vi "omni drive gyro.vi"(0 "Drive RefNum":T3={"DevStatus"={"status"=FALSE, "code"=0, "source"=""}, "Motors[]"=[], "Square Inputs"=FALSE, "Max Output"=1.0}, 1 "X Axis":dbl, 2 "Y Axis":dbl, 3 "Z Axis":dbl, 4 "Drive Mode":T1=enum."Arcade Drive", 5 "Center Motor":T4={"DeviceStatus"={"status"=FALSE, "code"=0, "source"=""}, "Type"=enum."PWM", "PWM"={"Controller"=enum."Controller 1", "PWM Channel"=enum."Invalid", "DeadBand"={"Name"="", "maxPositivePwm"=0, "minPositivePwm"=0, "centerPwm"=0, "maxNegativePwm"=0, "minNegativePwm"=0, "angularRange"=0}}, "CAN"={"Device Number"=0, "Control Mode"=enum."Percent VBus", "Semaphore"=refnum, "Max Vout"=12.0, "TalonSRX Control Mode"=enum."Percent VBus"}, "Invert"=FALSE, "TransformRef"=refnum, "InvTransformRef"=refnum}, 9 "Desired Angle":dbl) -> ()   [LabVIEW 2014]
uses:
  typedefs/drive mode.ctl
  <vilib>/Rock Robotics/WPI/RobotDrive/WPI_RobotDriveDevRef.ctl
  <vilib>/Rock Robotics/WPI/MotorControl/WPI_MotorControlDeviceRef.ctl
  <vilib>/Rock Robotics/WPI/MotorControl/WPI_MotorControlType.ctl
  <vilib>/Rock Robotics/SystemInterfaces/Typedef/FPGA_TypedefDigitalModule.ctl
  <vilib>/Rock Robotics/SystemInterfaces/DIO/FPGA_DIOPWMChannel.ctl
  <vilib>/Rock Robotics/WPI/PWM/WPI_PWMDeadband.ctl
  <vilib>/Rock Robotics/WPI/CAN/Jaguar/SubVIs/WPI_CANJaguar_ControlMode.ctl
  <vilib>/Rock Robotics/WPI/CAN/TalonSRX/WPI_CANTalonSRX_APIControlMode.ctl
  <vilib>/Rock Robotics/WPI/PWM/WPI_PWMTransform_ConPane.ctl
  typedefs/state machine/subStates.ctl
  global variables/devrefs.vi
  <vilib>/addons/control/pid/pid.llb/PID (DBL).vi
  <vilib>/Rock Robotics/WPI/RobotDrive/WPI_RobotDriveArcadeDrive_Standard(NoSaturation).vi
  global variables/dashboard data.vi
  <vilib>/addons/control/pid/NI_PID_pid.lvlib
panel:
  in  "Omni-Drive Tab Control":enum32{"Drive I/O", "PID", "Motor Controls"}(tab)
  in  "Spin Factor":dbl(slide) min=0.0 max=2.0 step=0.1 scale=0.0..2.0
  in  "PID Gains":T2={"proportional gain (Kc)"=0.0592, "integral time (Ti, min)"=0.0015, "derivative time (Td, min)"=0.0025} {"derivative time (Td, min)" step=0.0001 format="%.5f"; "integral time (Ti, min)" step=0.0001 format="%.5f"; "proportional gain (Kc)" step=0.0001 format="%.5f"}
  out "Gyro Temp °C":dbl
  out "Gyro Temp °F":dbl
  out "Setpoint Angle":dbl format="%#_6g°"
  out "Current Angle":dbl format="%#_g°"
  out "PID & Gyro Waveform Chart":cluster{"Angle":dbl, "output":dbl}(graph)
  out "Angular Rate":dbl
  # "Drive the Robot in Either Arcade Style or H-Drive Style"
  # "VI Inputs"
  # "OKish values rev1\nP: 0.00040\nI: 0.00100\nD: 0.00000\n\nPretty Good values\nP: 0.02\nI: 0.005\nD: 0.001\n\nBetter values?\nP: 0.0025\nI: 0.002\nD: 0.001\n\n0.009\n0.006"
  # "Thats a type def so you can't change it to the system\ncontrol otherwise it will no longer by linked to the typedef,\nand you can't re-link it"
  # "Temporary"
  # "Does this empty space make you feel uncomfortable?"
  # "Yes."
  # "I'm glad you feel that way."
  # "Note: Current Angle only updated in H-Drive, \nSetpoint updated in Arcade"
  # "°/sec"
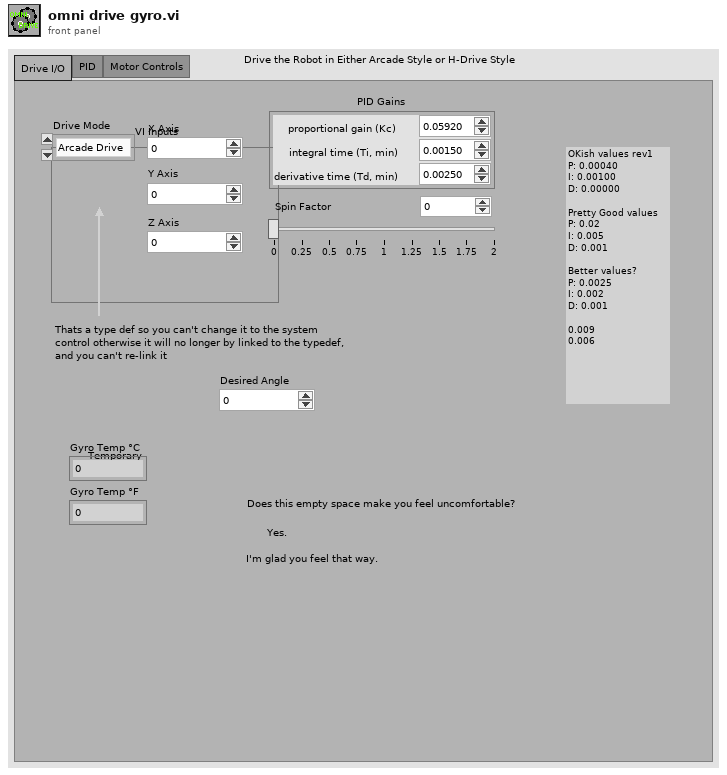
[diagram p1: front panel]
types:
  T1 = typedef "drive mode.ctl" = enum16{"Left/Right X/Y Control", "Arcade Drive", "H-Drive", "H-Drive Spin", "H-Drive PID", "Autonomous"}
  T2 = cluster{"proportional gain (Kc)":dbl, "integral time (Ti, min)":dbl, "derivative time (Td, min)":dbl}
  T3 = typedef "WPI_RobotDriveDevRef.ctl" = cluster{"DevStatus":errorcluster, "Motors[]":T4[], "Square Inputs":bool, "Max Output":dbl}
  T4 = typedef "WPI_MotorControlDeviceRef.ctl" = cluster{"DeviceStatus":errorcluster, "Type":T5, "PWM":cluster{"Controller":T6, "PWM Channel":T7, "DeadBand":T8}, "CAN":cluster{"Device Number":u8, "Control Mode":T9, "Semaphore":T10, "Max Vout":dbl, "TalonSRX Control Mode":T11}, "Invert":bool, "TransformRef":T12, "InvTransformRef":T12}
  T5 = typedef "WPI_MotorControlType.ctl" = enum16{"PWM", "CAN", "CANTalonSRX"}
  T6 = typedef "FPGA_TypedefDigitalModule.ctl" = enum16{"Controller 1"}
  T7 = typedef "FPGA_DIOPWMChannel.ctl" = enum8{"PWM 0", "PWM 1", "PWM 2", "PWM 3", "PWM 4", "PWM 5", "PWM 6", "PWM 7", "PWM 8", "PWM 9", "PWM MXP 0", "PWM MXP 1", "PWM MXP 2", "PWM MXP 3", "PWM MXP 4", "PWM MXP 5", "PWM MXP 6", "PWM MXP 7", "PWM MXP 8", "PWM MXP 9", "Invalid"}
  T8 = typedef "WPI_PWMDeadband.ctl" = cluster{"Name":string, "maxPositivePwm":i32, "minPositivePwm":i32, "centerPwm":i32, "maxNegativePwm":i32, "minNegativePwm":i32, "angularRange":u16}
  T9 = typedef "WPI_CANJaguar_ControlMode.ctl" = enum8{"Percent VBus", "Current", "Speed", "Position", "Voltage"}
  T10 = typedef "Semaphore RefNum" = refnum<k1>
  T11 = typedef "WPI_CANTalonSRX_APIControlMode.ctl" = enum8{"Percent VBus", "Speed", "Position", "Slave", "Unchanged / Invalid"}
  T12 = typedef "WPI_PWMTransform_ConPane.ctl" = refnum<vi>
  T13 = typedef "subStates.ctl" = enum16{"null", "wait", "driver control", "auto", "manual override", "hold position", "rotate", "test", "end"}
  T14 = typedef "WPI_GyroDevRef.ctl" = cluster{"DevStatus":errorcluster, "Analog Module":T15, "Analog Channel":T16, "Offset":dbl, "Gain (VoltsPerDegree/Second)":dbl}
  T15 = typedef "FPGA_TypedefAnalogModule.ctl" = enum16{"Controller 1"}
  T16 = typedef "FPGA_AIChannel.ctl" = enum8{"AI 0", "AI 1", "AI 2", "AI 3", "AI MXP 0", "AI MXP 1", "AI MXP 2", "AI MXP 3", "Invalid"}
  T17 = typedef "WPI_AnalogChannelDevRef.ctl" = cluster{"DevStatus":errorcluster, "Controller":T15, "Analog Channel":T16}
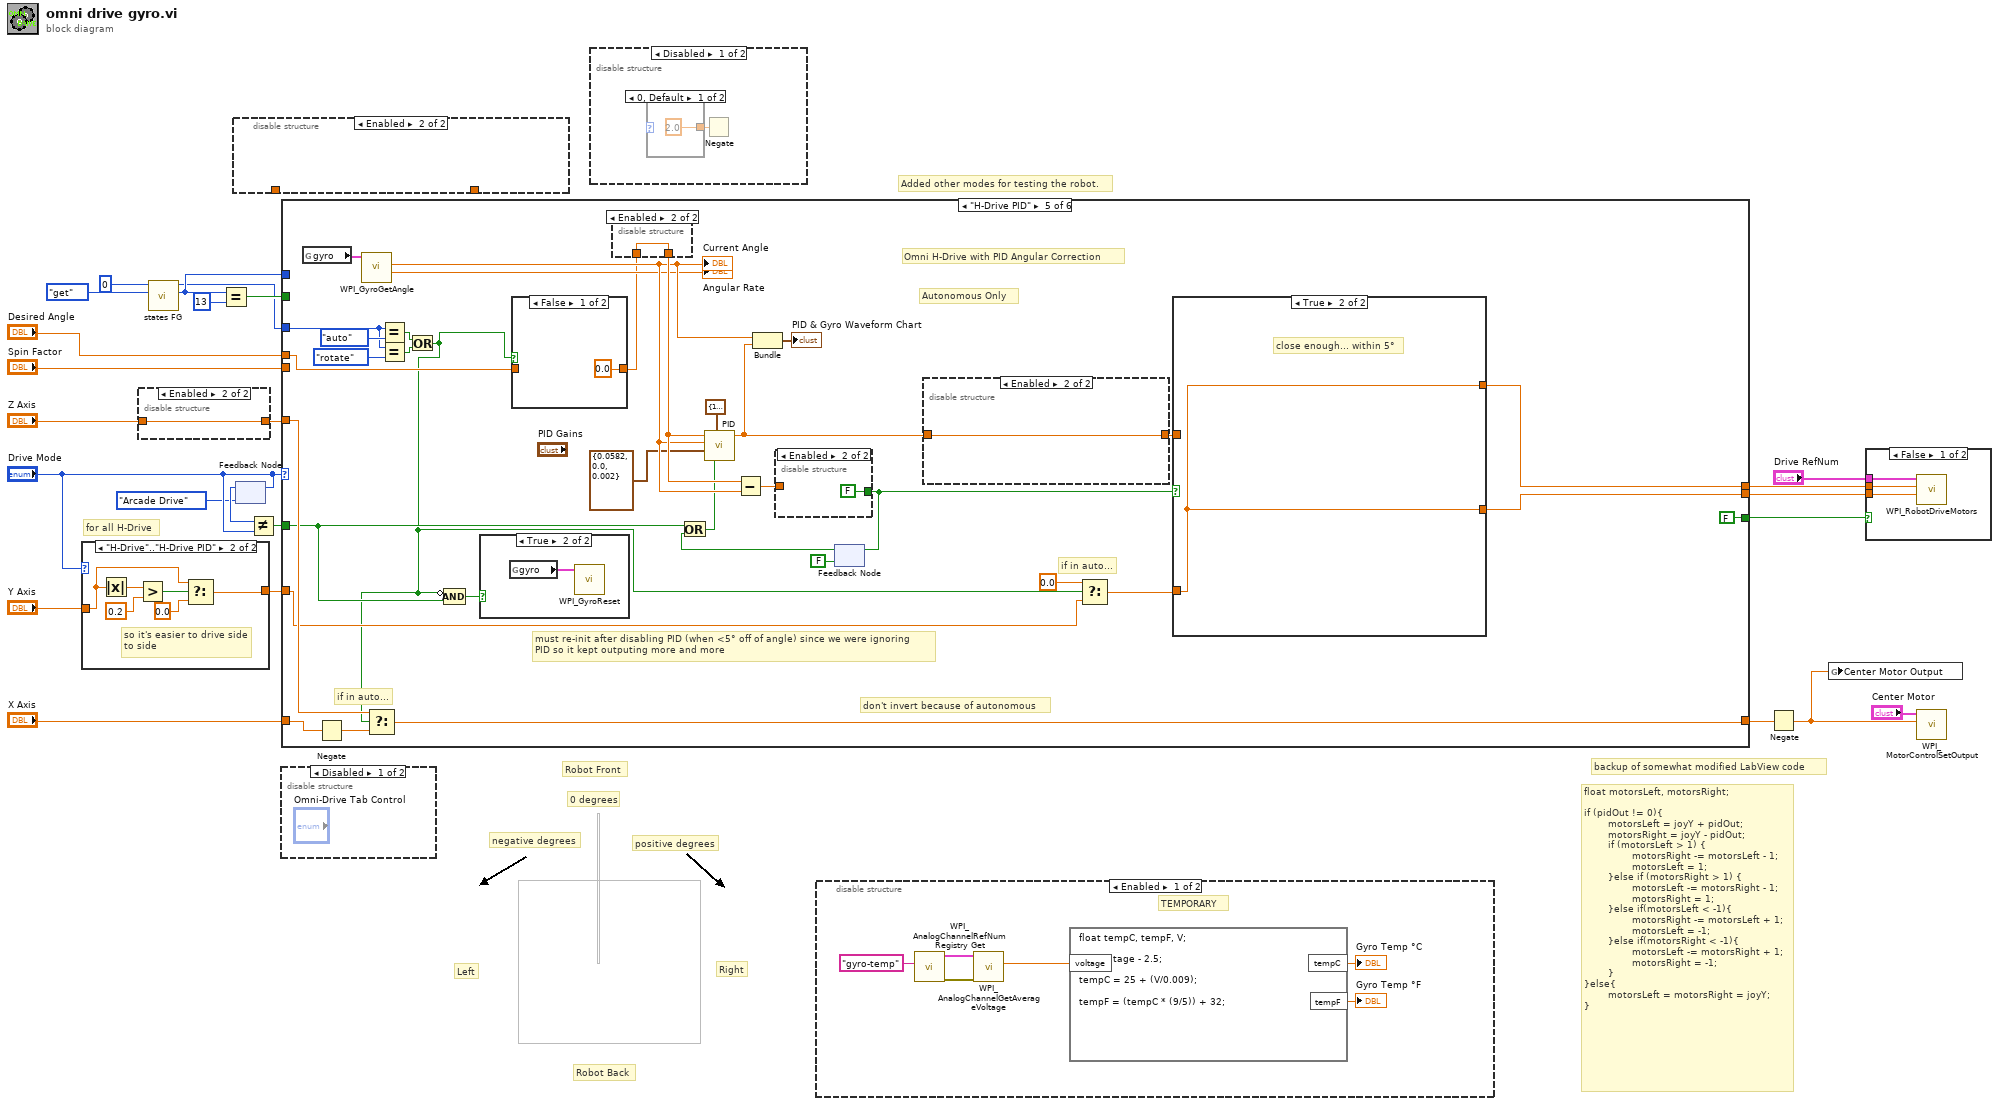
[diagram p0: block diagram]
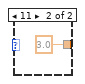
[diagram p2: hidden frame]
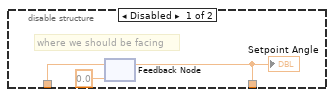
[diagram p4: hidden frame]
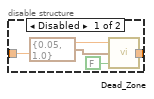
[diagram p7: hidden frame]
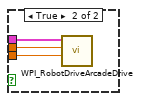
[diagram p9: hidden frame]
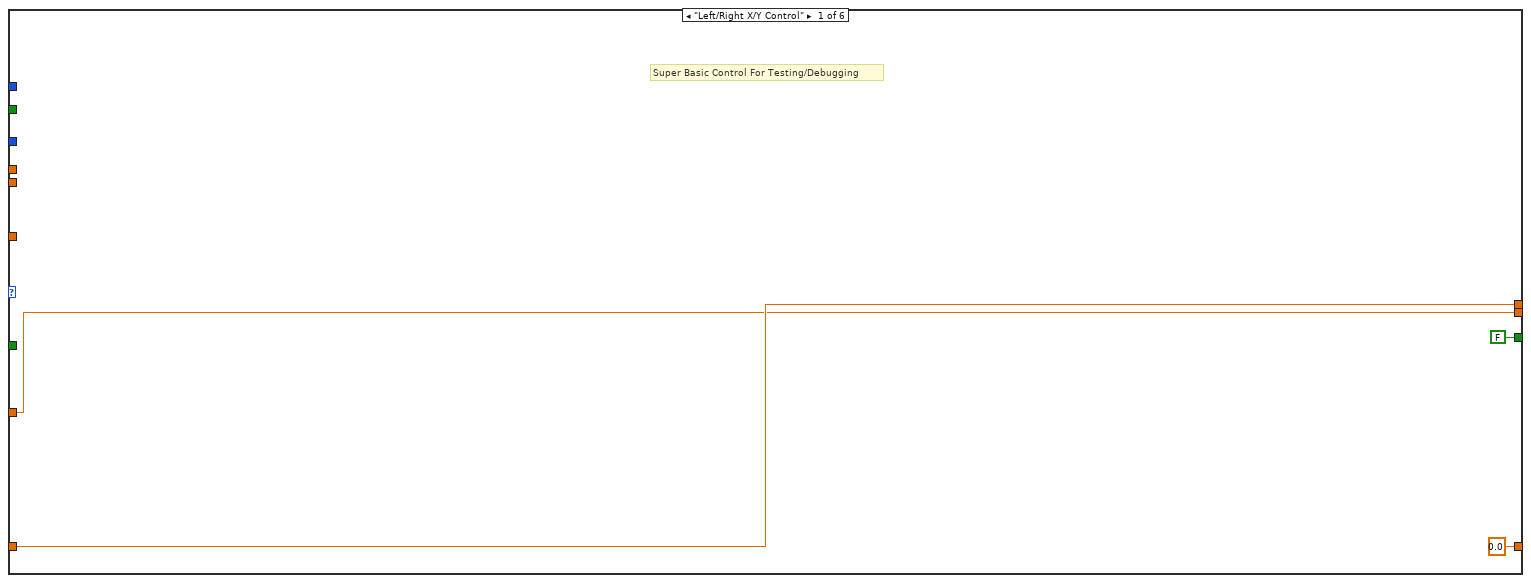
[diagram p10: hidden frame]
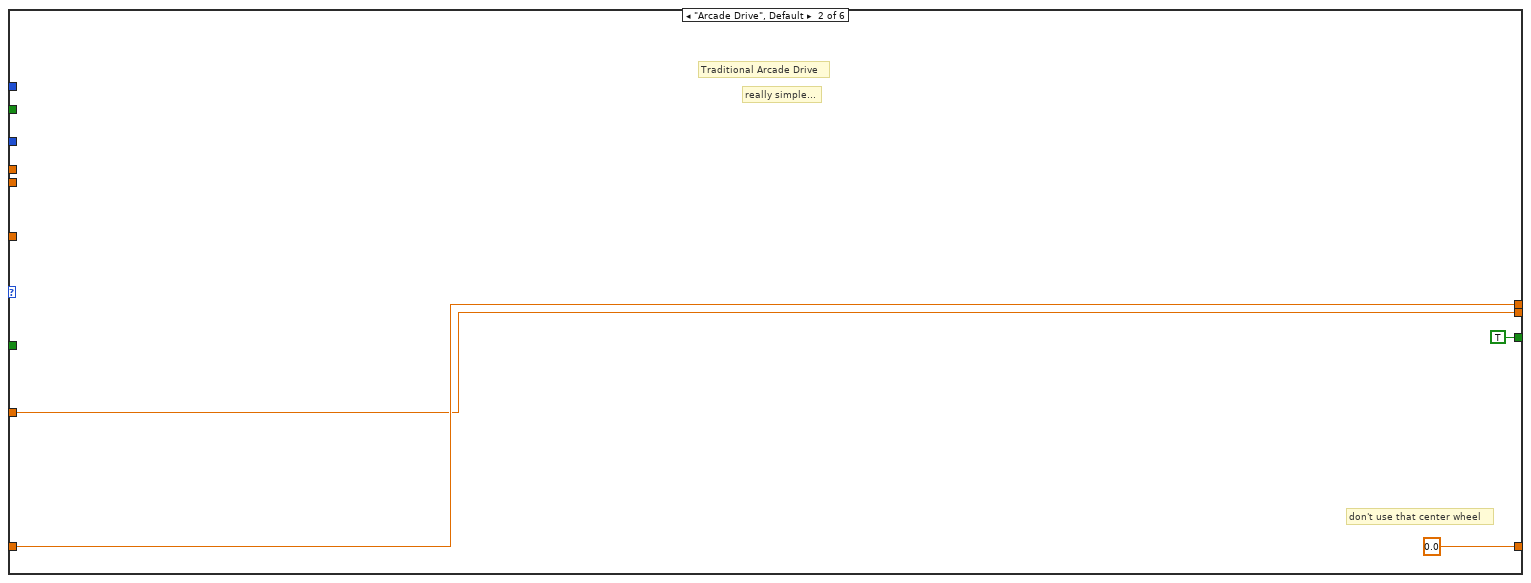
[diagram p11: hidden frame]
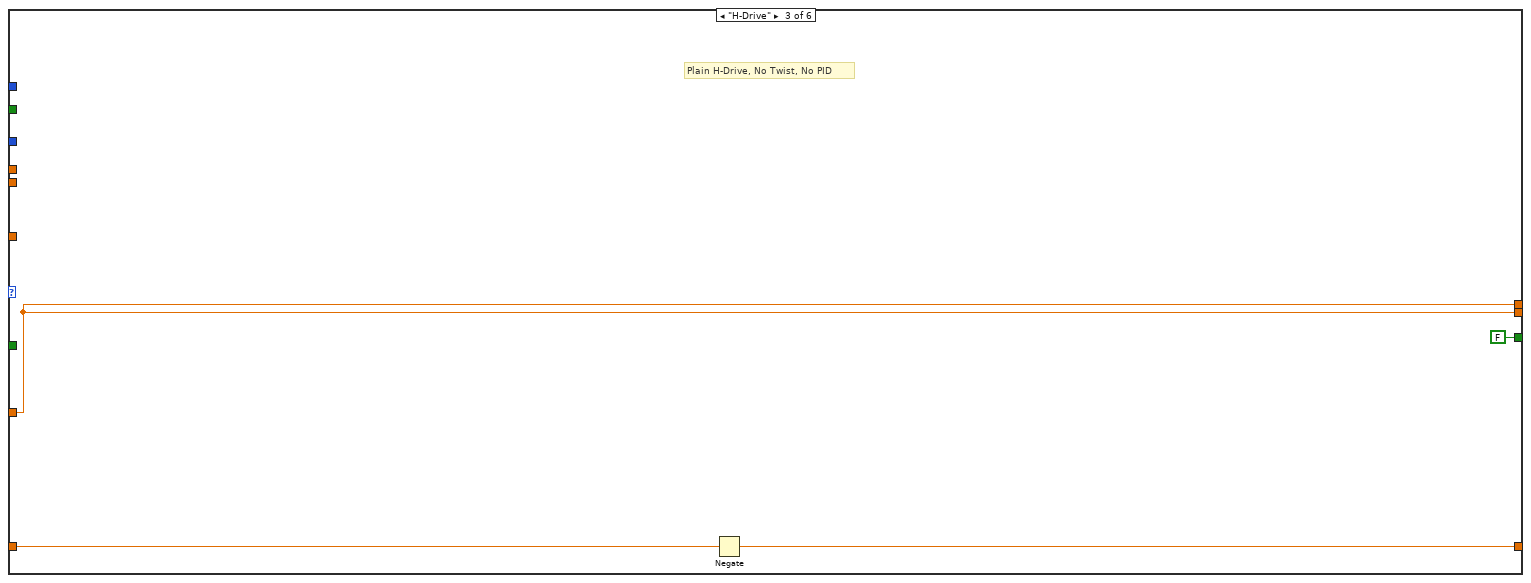
[diagram p12: hidden frame]
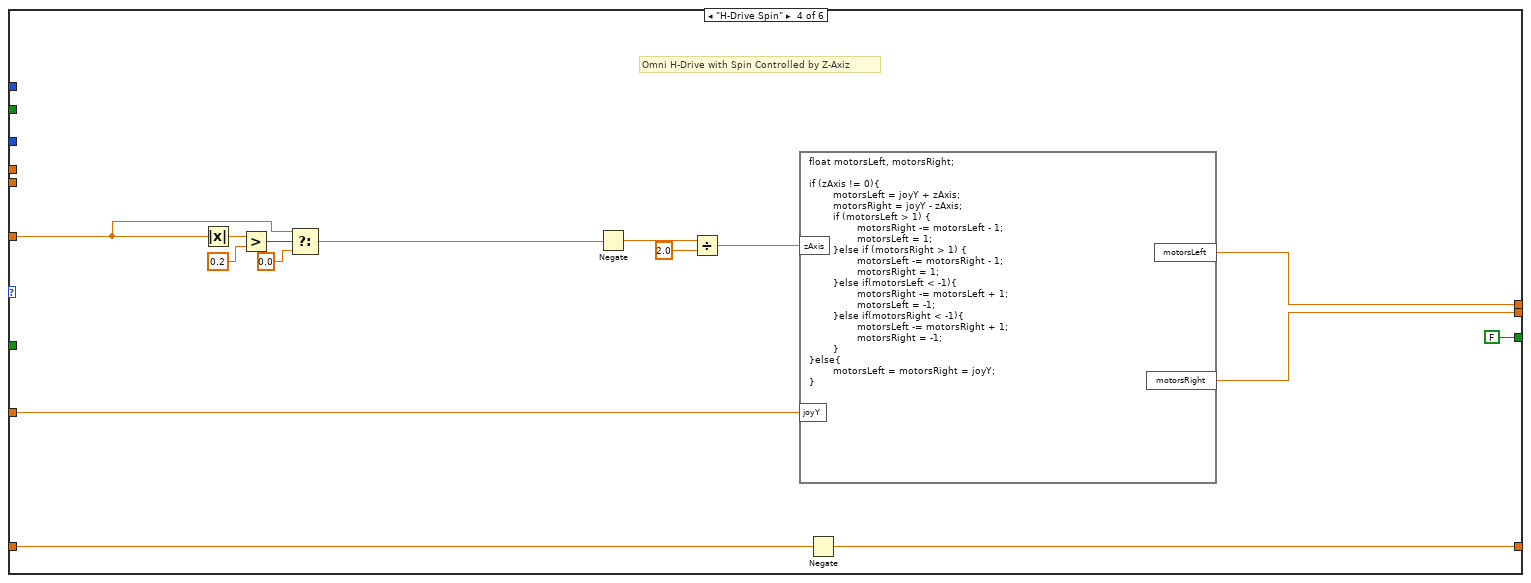
[diagram p13: hidden frame]
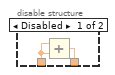
[diagram p14: hidden frame]
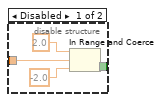
[diagram p17: hidden frame]
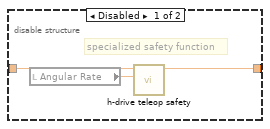
[diagram p18: hidden frame]
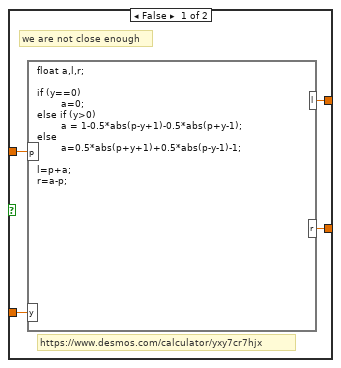
[diagram p19: hidden frame]
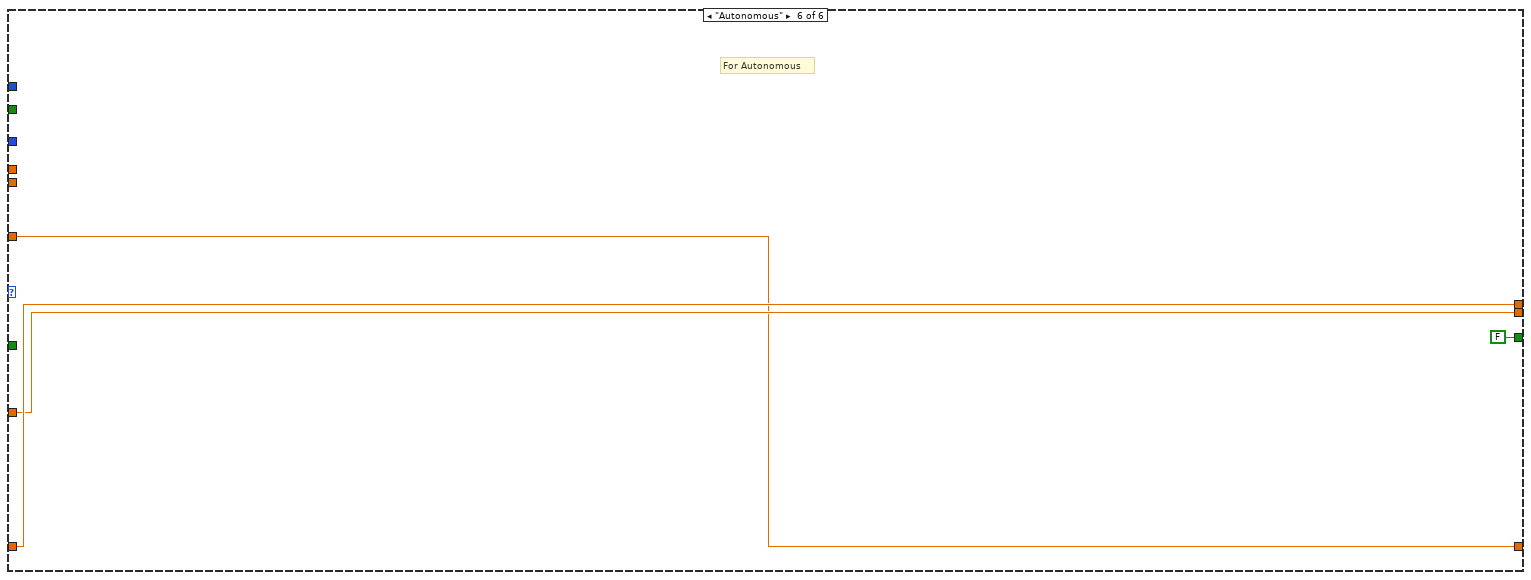
[diagram p20: hidden frame]
diagram:
  # "for all H-Drive"
  # "Added other modes for testing the robot."
  # "backup of somewhat modified LabView code"
  # "float motorsLeft, motorsRight;\n\nif (pidOut != 0){\n        motorsLeft = joyY + pidOut;\n        motorsRight = joyY - pidOut;\n        if (motorsLeft > 1) {\n                motorsRight -= motorsLeft - 1;\n                motorsLeft = 1;\n        }else if (motorsRight > 1) {\n                motorsLeft -= motorsRight - 1;\n                motorsRight = 1;\n        }else if(motorsLeft < -1){\n                motorsRight -= motorsLeft + 1;\n                motorsLeft = -1;\n        }else if(motorsRight < -1){\n                motorsLeft -= motorsRight + 1;\n                motorsRight = -1;\n        }\n}else{\n        motorsLeft = motorsRight = joyY;\n}"
  # "Robot Back"
  # "Right"
  # "Left"
  # "negative degrees"
  # "positive degrees"
  # "0 degrees"
  # "Robot Front"
  n1 = case shown="\"H-Drive\"..\"H-Drive PID\"" "Drive Mode" {
    tunnel: [w25 w26] -> w11
    tunnel: "Y Axis" -> [w25 w28]
    frame Default {
    }
    frame "H-Drive".."H-Drive PID" {
      # "so it's easier to drive side\nto side"
      n2 = Absolute Value(x=w28) -> (abs(x)=w31:dbl)
      n3 = Greater?(x=w31, y=0.2) -> (0:w29:bool)
      n4 = Select(t=w28, s=w29, f=0.0) -> (s? t:f=w26:dbl)
    }
  }
  n5 = disable-structure shown="Enabled" {
    disable-tunnel: [w35 w36] -> w13
    disable-tunnel: "Z Axis" -> [w34 w36]
    frame Disabled {
      n6 = call "Dead_Zone.vi"("Slope of 1"=FALSE, "Dead Zone and Limits"=cluster{dbl, dbl} {0.05, 1.0}, "Input"=w34) -> ("Output"=w35:dbl)  [unwired: 1 in]
    }
    frame Enabled {
    }
  }
  n7 = call "states FG.vi"("menu (get)"=enum16{"set", "get"}."get", "Loop ID"=0) -> ("state # out"=w3:i32, "subState out"=w2:T13)  [unwired: 6 in, 2 out]
  n8 = Equal?(x=w3, y=13) -> (x = y?=w5:bool)
  n9 = disable-structure shown="Enabled" {
    disable-tunnel: _ -> [w39 _]
    disable-tunnel: [w37 _] -> _
    frame Disabled {
      # "where we should be facing"
      n10 = feedback #1(0.0) -> (w37:dbl)
      n11 = feedback-in #1(w39) -> ()
      "Setpoint Angle" <- w39
    }
    frame Enabled {
    }
  }
  n12 = feedback-in #2("Drive Mode") -> ()
  n13 = feedback #2(drive_mode."Arcade Drive" ("Drive Mode")) -> (w17:T1)
  n14 = Not Equal?(x=w17, y="Drive Mode") -> (x != y?=w16:bool)
  n15 = case shown="\"H-Drive PID\"" "Drive Mode" {
    tunnel: [0.0 ("X Axis") 0.0 w48 w58 w79 w121] -> w14
    tunnel: [w42 w46 w50 w62 w85 w122] -> w23
    tunnel: [w43 w47 w50 w63 w86 w123] -> w22
    tunnel: "X Axis" -> [w43 w47 w49 w64 w78 w123]
    tunnel: w11 -> [w42 w46 w50 w65 w75 w122]
    tunnel: [FALSE TRUE FALSE FALSE FALSE FALSE] -> w20
    tunnel: w16 -> [_ _ _ _ w81 _]
    tunnel: w13 -> [_ _ _ w52 w82 w121]
    tunnel: "Spin Factor" -> [_ _ _ _ _ _]
    tunnel: w5 -> [_ _ _ _ _ _]
    tunnel: w3 -> [_ _ _ _ _ _]
    tunnel: w2 -> [_ _ _ _ w71 _]
    tunnel: "Desired Angle" -> [_ _ _ _ w74 _]
    frame "Left/Right X/Y Control" {
      # "Super Basic Control For Testing/Debugging"
    }
    frame "Arcade Drive", Default {
      # "really simple..."
      # "don't use that center wheel"
      # "Traditional Arcade Drive"
    }
    frame "H-Drive" {
      # "Plain H-Drive, No Twist, No PID"
      n16 = Negate(x=w49) -> (-x=w48:dbl)
    }
    frame "H-Drive Spin" {
      # "Omni H-Drive with Spin Controlled by Z-Axiz"
      n17 = Absolute Value(x=w52) -> (abs(x)=w54:dbl)
      n18 = Greater?(x=w54, y=0.2) -> (0:w56:bool)
      n19 = Select(t=w52, s=w56, f=0.0) -> (s? t:f=w53:dbl)
      n20 = Negate(x=w53) -> (-x=w59:dbl)
      n21 = Divide(x=w59, y=2.0 ("x")) -> (x/y=w61:dbl)
      n22 = formula code="float motorsLeft, motorsRight;\n\nif (zAxis != 0){\n        motorsLeft = joyY + zAxis;\n        motorsRight = joyY - zAxis;\n        if (motorsLeft > 1) {\n                motorsRight -= motorsLeft - 1;\n                motorsLeft = 1;\n        }else if (motorsRight > 1) {\n                motorsLeft -= motorsRight - 1;\n                motorsRight = 1;\n        }else if(motorsLeft < -1){\n                motorsRight -= motorsLeft + 1;\n                motorsLeft = -1;\n        }else if(motorsRight < -1){\n                motorsLeft -= motorsRight + 1;\n                motorsRight = -1;\n        }\n}else{\n        motorsLeft = motorsRight = joyY;\n}"("zAxis"=w61, "joyY"=w65) -> ("motorsLeft"=w63:dbl, "motorsRight"=w62:dbl)
      n23 = Negate(x=w64) -> (-x=w58:dbl)
    }
    frame "H-Drive PID" {
      # "if in auto..."
      # "if in auto..."
      # "don't invert because of autonomous"
      # "Autonomous Only"
      # "must re-init after disabling PID (when <5° off of angle) since we were ignoring\nPID so it kept outputing more and more"
      # "Omni H-Drive with PID Angular Correction"
      n24 = global read "devrefs.vi" "gyro"() -> (w96:T14)
      n25 = Negate(x=w78) -> (-x=w67:dbl)
      n26 = call <vilib>:"WPI_GyroGetAngle.vi"("GyroDevRef"=w96) -> ("Angular Rate"=→"Angular Rate":dbl, "Angle"=w99:dbl)  [unwired: 7 in, 2 out]
      "Current Angle" <- w99
      n27 = Equal?(x=w71, y=subStates."auto") -> (x = y?=w69:bool)
      n28 = Equal?(x=w71, y=subStates."rotate") -> (x = y?=w70:bool)
      n29 = Or(x=w69, y=w70) -> (x .or. y?=w68:bool)
      n30 = Select(t=w82, s=w68, f=w67) -> (s? t:f=w79:dbl)
      n31 = Compound Arithmetic op=AND(invert w68, w81) -> (w80:bool)
      n32 = case shown="True" w80 {
        frame False {
        }
        frame True {
          n33 = global read "devrefs.vi" "gyro"() -> (w104:T14)
          n34 = call <vilib>:"WPI_GyroReset.vi"("GyroDevRef"=w104) -> ()  [unwired: 9 in, 2 out]
        }
      }
      n35 = case shown="False" w68 {
        tunnel: [0.0 w106] -> w84
        tunnel: w74 -> [_ w106]
        frame False {
        }
        frame True {
        }
      }
      n36 = disable-structure shown="Enabled" {
        disable-tunnel: [w102 w103] -> w100
        disable-tunnel: w84 -> [w101 w103]
        frame Disabled {
          n37 = Add(x=w101, y=w101) -> (x+y=w102:dbl)
        }
        frame Enabled {
        }
      }
      n38 = Subtract(x=w100, y=w99) -> (x-y=w91:dbl)
      n39 = disable-structure shown="Enabled" {
        disable-tunnel: [w110 FALSE] -> w94
        disable-tunnel: w91 -> [w109 _]
        frame Disabled {
          n40 = In Range and Coerce(upper limit=2.0, x=w109, lower limit=-2.0 ("upper limit")) -> (In Range?=w110:bool)  [unwired: 1 out]
        }
        frame Enabled {
        }
      }
      n41 = feedback #3(FALSE) -> (w90:bool)
      n42 = Or(x=w81, y=w90) -> (x .or. y?=w93:bool)
      n43 = call-poly <vilib>:"PID.vi"("reinitialize? (F)"=w93, "output range"=cluster{"output high":dbl, "output low":dbl} {"output high"=1.0, "output low"=-1.0}, "PID gains"=T2 {"proportional gain (Kc)"=0.0582, "integral time (Ti, min)"=0.0, "derivative time (Td, min)"=0.002} ("PID Gains 2"), "process variable"=w99, "setpoint"=w100) -> ("output"=w88:dbl)  [unwired: 5 in, 1 out]
      n44 = Bundle("Angle"=w99, "output"=w88) -> (→"PID & Gyro Waveform Chart":cluster{"Angle":dbl, "output":dbl})  [unwired: 1 in]
      n45 = feedback-in #3(w94) -> ()
      n46 = disable-structure shown="Enabled" {
        disable-tunnel: w88 -> [w114 w115]
        disable-tunnel: [w113 w115] -> w87
        frame Disabled {
          # "specialized safety function"
          n47 = local read "Angular Rate"() -> (w112:dbl)
          n48 = call "h-drive teleop safety.vi"("Gyro Angular Rate"=w112, "Input"=w114) -> ("Output"=w113:dbl)  [unwired: 9 in]
        }
        frame Enabled {
        }
      }
      n49 = Select(t=0.0, s=w68, f=w75) -> (s? t:f=w77:dbl)
      n50 = case shown="True" w94 {
        tunnel: w87 -> [w117 _]
        tunnel: [w119 w120] -> w85
        tunnel: [w118 w120] -> w86
        tunnel: w77 -> [w116 w120]
        frame False {
          # "https://www.desmos.com/calculator/yxy7cr7hjx"
          # "we are not close enough"
          n51 = formula code="float a,l,r;\n\nif (y==0) \n        a=0;\nelse if (y>0) \n        a = 1-0.5*abs(p-y+1)-0.5*abs(p+y-1);\nelse \n        a=0.5*abs(p+y+1)+0.5*abs(p-y-1)-1;\n\nl=p+a;\nr=a-p;"("p"=w117, "y"=w116) -> ("l"=w118:dbl, "r"=w119:dbl)
        }
        frame True {
          # "close enough... within 5°"
        }
      }
    }
    frame "Autonomous" {
      # "For Autonomous"
    }
  }
  n52 = disable-structure shown="Disabled" {
    frame Disabled {
    }
    frame Enabled {
    }
  }
  n53 = disable-structure shown="Disabled" {
    frame Disabled {
      n54 = case shown="0, Default" {
        selector: _ -> [_ _]
        tunnel: [2.0 3.0] -> w125
        frame 0, Default {
        }
        frame 11 {
        }
      }
      n55 = Negate(x=w125) -> ()  [unwired: 1 out]
    }
    frame Enabled {
    }
  }
  n56 = disable-structure shown="Enabled" {
    frame Enabled {
      # "TEMPORARY"
      n57 = call <vilib>:"WPI_AnalogChannelRefNum Registry Get.vi"("refnum name"="gyro-temp") -> ("error out"=w133:errorcluster, "AIDeviceRef"=w132:T17)  [unwired: 9 in]
      n58 = call <vilib>:"WPI_AnalogChannelGetAverageVoltage.vi"("error in (no error)"=w133, "AIDeviceRef"=w132) -> ("Voltage"=w130:dbl)  [unwired: 7 in, 2 out]
      n59 = formula code="float tempC, tempF, V;\n\nV = voltage - 2.5;\n\ntempC = 25 + (V/0.009);\n\ntempF = (tempC * (9/5)) + 32;"("voltage"=w130) -> ("tempC"=→"Gyro Temp °C":dbl, "tempF"=→"Gyro Temp °F":dbl)
    }
    frame Disabled {
    }
  }
  n60 = Negate(x=w14) -> (-x=w8:dbl)
  n61 = global write "dashboard data.vi" "Center Motor Output"(w8) -> ()
  n62 = case shown="False" w20 {
    tunnel: "Drive RefNum" -> [w136 w139]
    tunnel: w23 -> [w134 w138]
    tunnel: w22 -> [w135 w137]
    frame False {
      n63 = call <vilib>:"WPI_RobotDriveMotors.vi"("RightSpeed"=w134, "LeftSpeed"=w135, "RobotDriveDevRef"=w136) -> ()  [unwired: 6 in, 3 out]
    }
    frame True {
      n64 = call-poly <vilib>:"WPI_RobotDriveArcadeDrive.vi"("Y axis value"=w138, "X axis value"=w137, "RobotDriveDevRef"=w139) -> ()  [unwired: 6 in, 3 out]
    }
  }
  n65 = call <vilib>:"WPI_MotorControlSetOutput.vi"("Output"=w8, "MotorControlDevRef"="Center Motor") -> ()  [unwired: 7 in, 3 out]
